vi "RSZVB Get User Defined Preset State.vi"(8 "error in (no error)":errorcluster {"code" format="%.0x"}, 11 "VISA session":refnum<visa-resource-name>) -> (0 "error out":errorcluster {"code" format="%.0x"}, 1 "User Defined Preset":bool, 3 "dup VISA session":refnum<visa-resource-name>)   [LabVIEW 2011]
doc: "This VI returns a state of the user-defined preset.\n\nRemote-control command(s):\nSYSTem:PRESet:USER[:STATe]?"
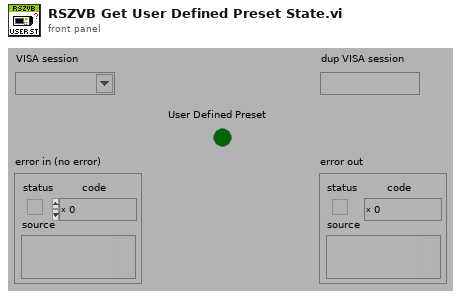
[diagram p1: front panel]
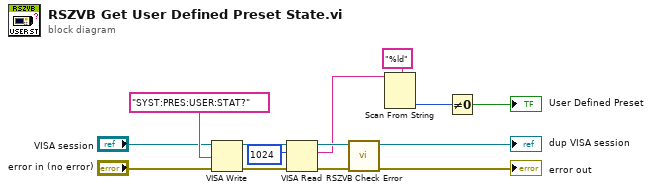
[diagram p0: block diagram]
diagram:
  n1 = VISA Write(VISA resource name="VISA session", write buffer="SYST:PRES:USER:STAT?", error in (no error)="error in (no error)") -> (VISA resource name out=w12:refnum<visa-resource-name>, error out=w14:errorcluster)  [unwired: 1 out]
  n2 = VISA Read(VISA resource name=w12, byte count=u32 1024 ("byte count (0)"), error in (no error)=w14) -> (VISA resource name out=w11:refnum<visa-resource-name>, read buffer=w2:string, error out=w10:errorcluster)  [unwired: 1 out]
  n3 = call "RSZVB Check Error.vi"("error in (no error)"=w10, "VISA session"=w11) -> ("error out"=→"error out":errorcluster, "dup VISA session"=→"dup VISA session":refnum<visa-resource-name>)  [unwired: 8 in]
  n4 = Scan From String(format string="%ld", input string=w2) -> (output 1=w1:i32)  [unwired: 3 in, 3 out]
  n5 = Not Equal To 0?(x=w1) -> (x != 0?=→"User Defined Preset":bool)
